vi "Conteggio numero interventi su un pulsante - Shift example.vi"(1 "Delay":u32=1000, 2 "stop":bool, 3 "switch":bool) -> (0 "n° inter.":i32)   [LabVIEW 2012]
doc: "© Copyright M. Ferrari 2000\n Shift register example 2"
panel:
  out "N iter -1":dbl format="%.2f"
  out "N iter -2":dbl format="%.2f"
  # "CONTATEGGIO DEL N° DI INTERVENTI su UN PULSANTE"
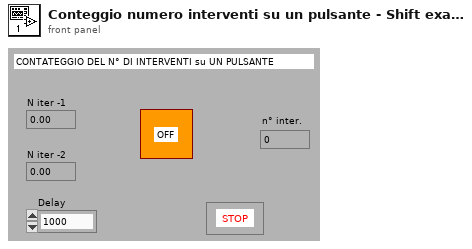
[diagram p1: front panel]
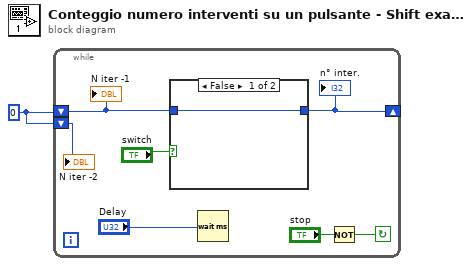
[diagram p0: block diagram]
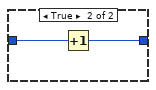
[diagram p2: hidden frame]
diagram:
  w1 = 0
  n1 = while {
    shift-right: [w3] -> _
    shift-left: w1 -> [w6]
    shift-left: w1 -> [w2]
    stop <- w7 continue-if-true
    n2 = case shown="False" "switch" {
      tunnel: w6 -> [w9 w11]
      tunnel: [w9 w10] -> w3
      frame False {
      }
      frame True {
        n3 = Increment(x=w11) -> (x+1=w10:i32)
      }
    }
    "n° inter." <- w3
    n4 = Wait (ms)(milliseconds to wait="Delay") -> ()  [unwired: 1 out]
    n5 = Not(x="stop") -> (.not. x?=w7:bool)
    "N iter -2" <- w2
    "N iter -1" <- w6
  }
